vi "Generate Name-Value Pair Array.vi"(11 "Name-Value Pair JSON":string) -> (3 "Name-Value Pairs":T1[](array[typedef]))   [LabVIEW 2015, in "NI_Azure_JSON Parsing.lvlib"]
uses:
  NI_Azure_JSON Parsing.lvlib
  Name Value Pair.ctl
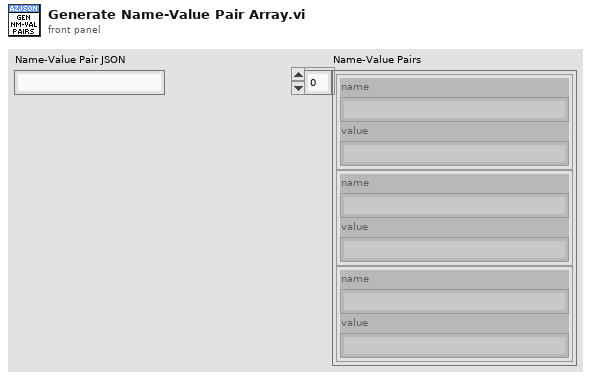
[diagram p1: front panel]
types:
  T1 = typedef "NI_Azure_JSON Parsing.lvlib/Name Value Pair.ctl" = cluster{"name":string, "value":string}
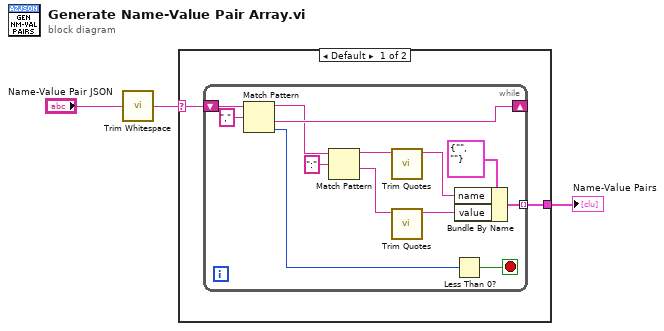
[diagram p0: block diagram]
diagram:
  n1 = call <vilib>:"Trim Whitespace.vi"("string"="Name-Value Pair JSON") -> ("trimmed string"=w1:string)  [unwired: 1 in]
  n2 = case shown="Default" w1 {
    selector: w1 -> [w4 _]
    tunnel: [w5 _] -> w2
    frame Default {
      n3 = while {
        shift-right: [w13] -> _
        shift-left: w4 -> [w18]
        tunnel: [w16] -> w5 mode=indexing
        stop <- w14 stop-if-true
        n4 = Match Pattern(string=w18, regular expression=",") -> (before substring=w12:string, after substring=w13:string, offset past match=w15:i32)  [unwired: 1 in, 1 out]
        n5 = Match Pattern(string=w12, regular expression=":" ("search string/char (-)")) -> (before substring=w10:string, after substring=w7:string)  [unwired: 1 in, 2 out]
        n6 = call "Trim Quotes.vi"("String"=w10) -> ("String without Quotes"=w9:string)  [unwired: 9 in, 1 out]
        n7 = call "Trim Quotes.vi"("String"=w7) -> ("String without Quotes"=w8:string)  [unwired: 9 in, 1 out]
        n8 = Less Than 0?(x=w15) -> (x < 0?=w14:bool)
        n9 = Bundle By Name(cluster=T1 {"name"="", "value"=""} ("Name Value Pair"), "name"=w9, "value"=w8) -> (w16:T1)
      }
    }
    frame "" {
    }
  }
  "Name-Value Pairs" <- w2
